vi "Handle Player.vi"(6 "Move Queue Element":T1, 7 "Move in":T4={"InPlayPos Dict"=variant(i32[] [])}, 8 "error in (no error)":errorcluster, 11 "Maze 2.0 in":refnum<class "SquareBattle.lvclass">) -> (0 "error out":errorcluster, 3 "Maze 2.0 out":refnum<class "SquareBattle.lvclass">, 5 "Move out":T4={"InPlayPos Dict"=variant(i32[] [])})   [LabVIEW 2014, in "SquareBattle.lvclass"]
uses:
  SquareBattle.lvclass
  Move State Cluster.ctl
  Move Queue Element Cluster.ctl
  Runner/Runner.lvclass
  Action Enum.ctl
  Direction Enum.ctl
  SquareBattle.lvclass/SquareBattle.ctl
  Runner Cluster.ctl
panel:
  # "NOTICE - YOU MUST NOT REMOVE THIS NOTICE. PER THE FOLLOWING LICENSE, YOU MAY REPRODUCE THIS SOFTWARE PROVIDED YOU FOLLOW THE TERMS\nOF THE LICENSE.\n\n---BEGIN BSD LICENSE (http://opensource.org/licenses/BSD-2-Clause)---\nCopyright (c) 2015, Endigit, Inc. <robert@endigit.com>\nAll rights reserved.\n\nRedistribution and use in source and binary forms, with or without modification, are permitted provided that the following conditions are met:\n\n1. Redistributions of source code must retain the above copyright notice, this list of conditions and the following disclaimer.\n\n2. Redistributions in binary form must reproduce the above copyright notice, this list of conditions and the following disclaimer in the documentation and/or other \nmaterials provided with the distribution.\n\nTHIS SOFTWARE IS PROVIDED BY THE COPYRIGHT HOLDERS AND CONTRIBUTORS \"AS IS\" AND ANY EXPRESS OR IMPLIED WARRANTIES, INCLUDING, BUT NOT \nLIMITED TO, THE IMPLIED WARRANTIES OF MERCHANTABILITY AND FITNESS FOR A PARTICULAR PURPOSE ARE DISCLAIMED. IN NO EVENT SHALL THE COPYRIGHT \nHOLDER OR CONTRIBUTORS BE LIABLE FOR ANY DIRECT, INDIRECT, INCIDENTAL, SPECIAL, EXEMPLARY, OR CONSEQUENTIAL DAMAGES (INCLUDING, BUT NOT \nLIMITED TO, PROCUREMENT OF SUBSTITUTE GOODS OR SERVICES; LOSS OF USE, DATA, OR PROFITS; OR BUSINESS INTERRUPTION) HOWEVER CAUSED AND ON \nANY THEORY OF LIABILITY, WHETHER IN CONTRACT, STRICT LIABILITY, OR TORT (INCLUDING NEGLIGENCE OR OTHERWISE) ARISING IN ANY WAY OUT OF THE USE \nOF THIS SOFTWARE, EVEN IF ADVISED OF THE POSSIBILITY OF SUCH DAMAGE.\n---END BSD LICENSE---"
  # "What information:\n\nfor in play squares:\nID of players in square\nIs attacked."
  # "What information:\n\nfor in play squares:\nID of players in square\nIs attacked."
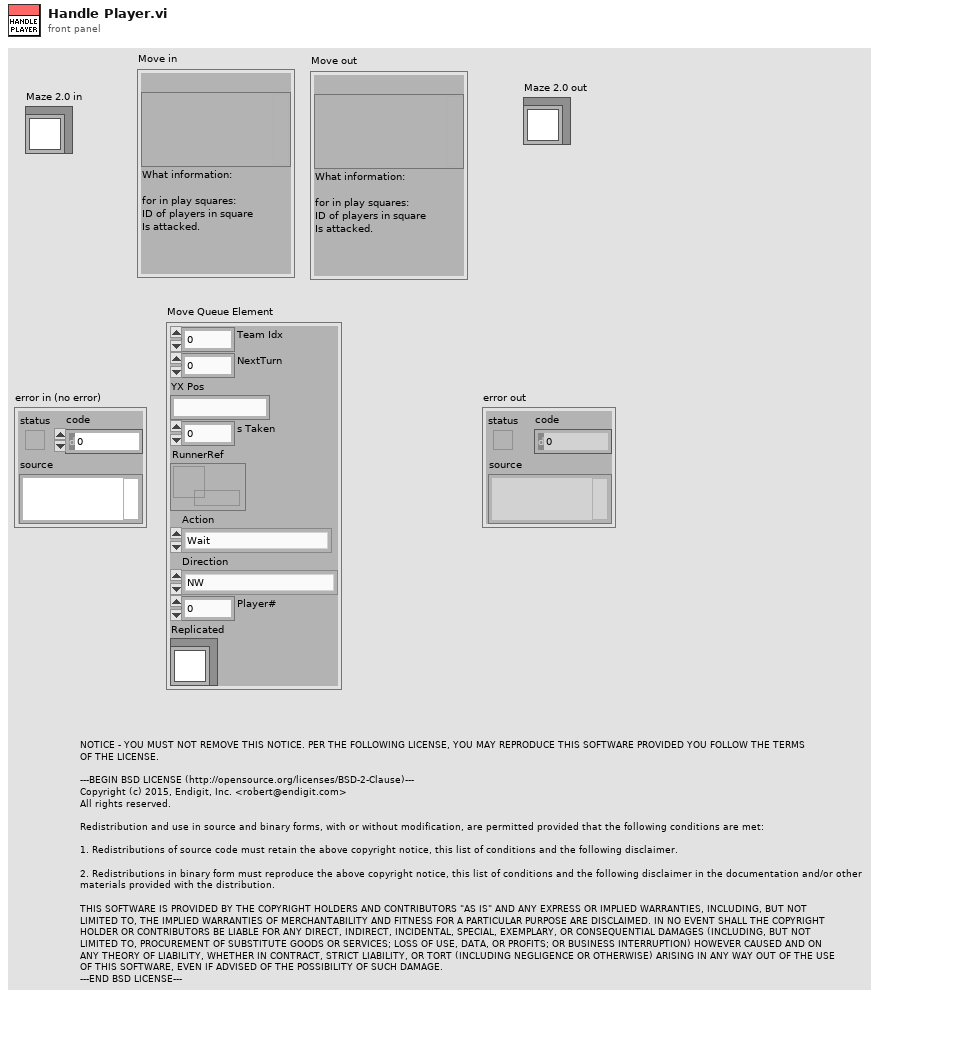
[diagram p1: front panel]
types:
  T1 = typedef "SquareBattle.lvclass/Move Queue Element Cluster.ctl" = cluster{"Team Idx":i32, "NextTurn":u32, "YX Pos":string, "s Taken":dbl, "RunnerRef":refnum<data-value>, "Action":T2, "Direction":T3, "Player#":i32, "Replicated":refnum<class "Runner.lvclass">}
  T2 = typedef "SquareBattle.lvclass/Action Enum.ctl" = enum16{"Wait", "Move", "Attack", "Replicate"}
  T3 = typedef "SquareBattle.lvclass/Direction Enum.ctl" = enum16{"NW", "N", "NE", "E", "SE", "S", "SW", "W"}
  T4 = typedef "SquareBattle.lvclass/Move State Cluster.ctl" = cluster{"InPlayPos Dict":variant}
  T5 = typedef "SquareBattle.lvclass/Runner Cluster.ctl" = cluster{"Attacked?":bool, "RunnerRef":refnum<data-value>, "TeamIdx":i32, "Player #":i32, "NextPlay":u32}
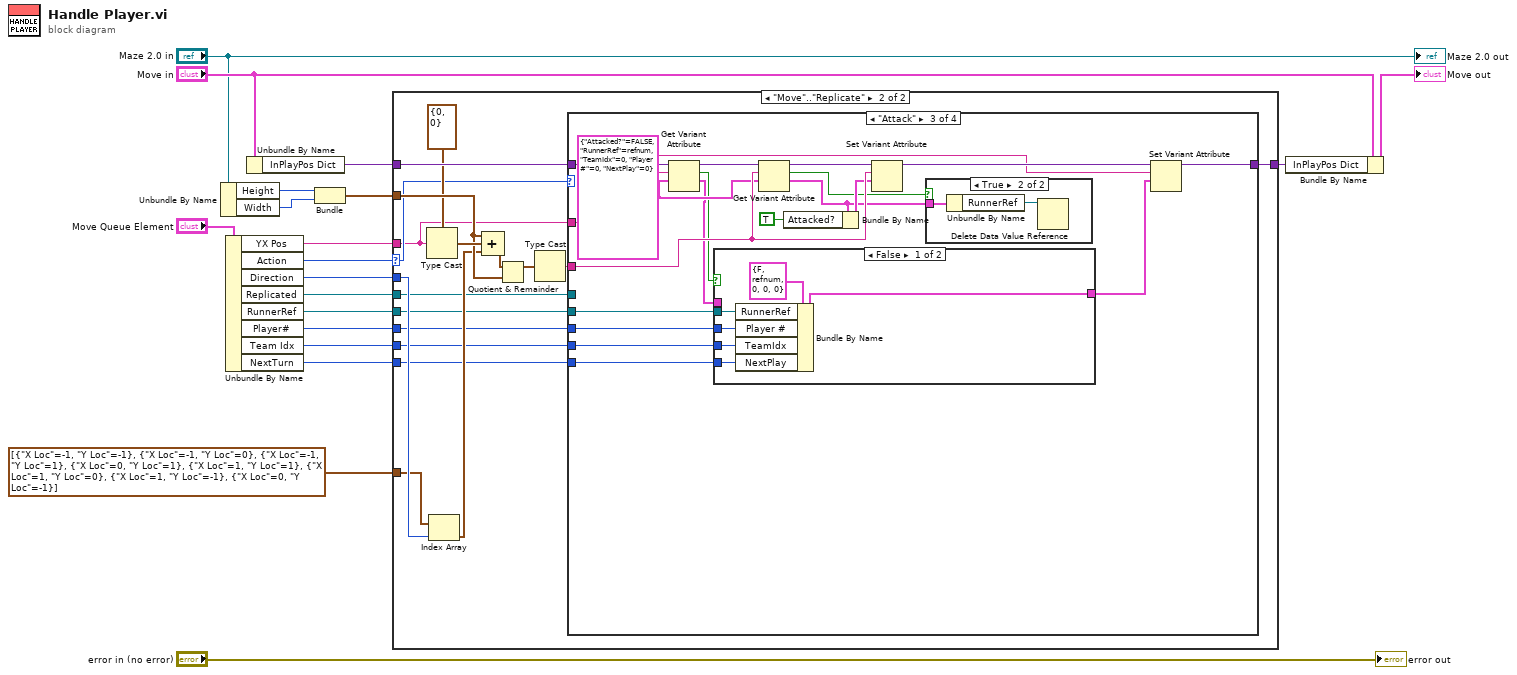
[diagram p0: block diagram]
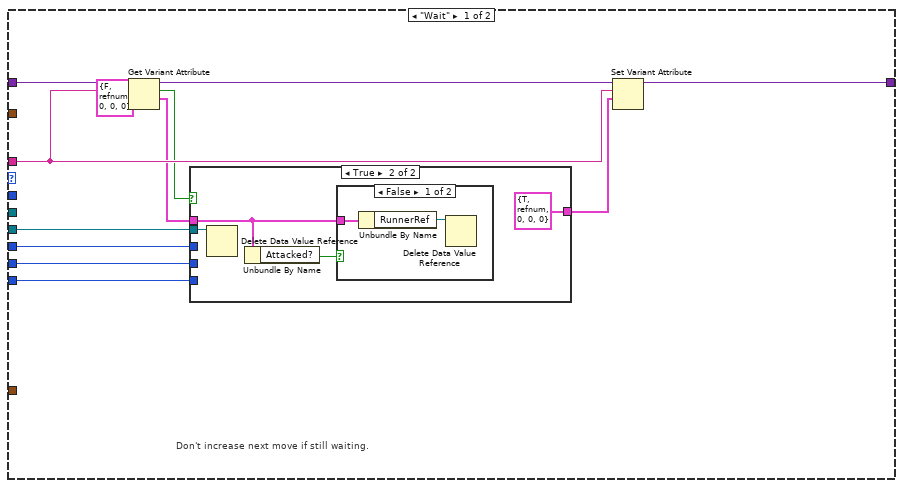
[diagram p2: hidden frame]
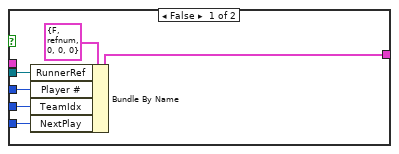
[diagram p3: hidden frame]
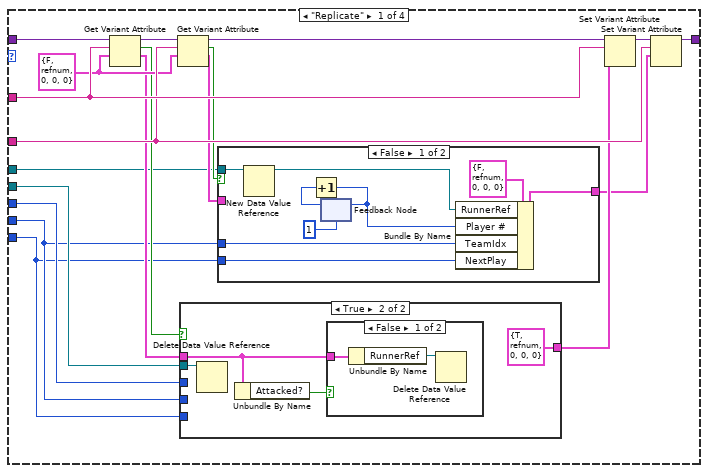
[diagram p5: hidden frame]
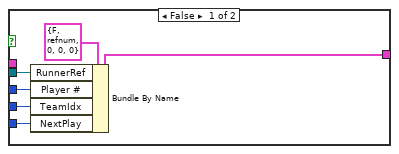
[diagram p6: hidden frame]
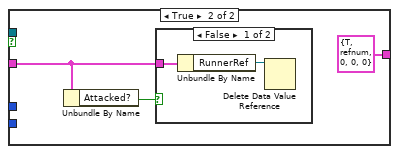
[diagram p8: hidden frame]
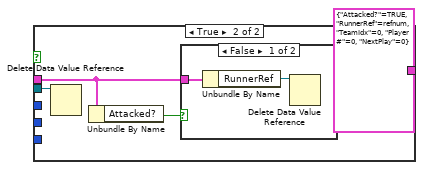
[diagram p12: hidden frame]
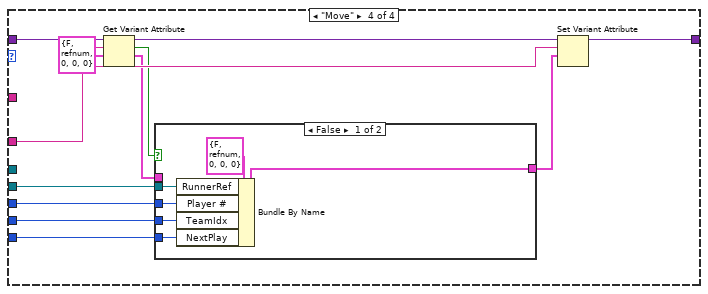
[diagram p14: hidden frame]
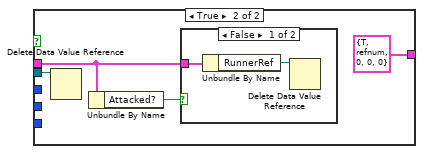
[diagram p15: hidden frame]
diagram:
  n1 = Unbundle By Name("Maze 2.0 in") -> ("Height"=w9:i32, "Width"=w8:i32)
  n2 = Unbundle By Name("Move Queue Element") -> ("YX Pos"=w13:string, "Action"=w12:T2, "Direction"=w16:T3, "Replicated"=w15:refnum<class "Runner.lvclass">, "RunnerRef"=w5:refnum<data-value>, "Player#"=w4:i32, "Team Idx"=w2:i32, "NextTurn"=w1:u32)
  n3 = Unbundle By Name("Move in") -> ("InPlayPos Dict"=w14:variant)
  n4 = Bundle("Height"=w9, "Width"=w8) -> (w7:cluster{"Height":i32, "Width":i32})  [unwired: 1 in]
  n5 = case shown="\"Move\"..\"Replicate\"" w12 {
    selector: w12 -> [_ w51]
    tunnel: w16 -> [_ w55]
    tunnel: w15 -> [_ w47]
    tunnel: w14 -> [w31 w61]
    tunnel: w13 -> [w24 w50]
    tunnel: w2 -> [w30 w49]
    tunnel: [w28 w46] -> w11
    tunnel: w7 -> [_ w57]
    tunnel: cluster{"X Loc":i32, "Y Loc":i32}[] [{"X Loc"=-1, "Y Loc"=-1}, {"X Loc"=-1, "Y Loc"=0}, {"X Loc"=-1, "Y Loc"=1}, {"X Loc"=0, "Y Loc"=1}, {"X Loc"=1, "Y Loc"=1}, {"X Loc"=1, "Y Loc"=0}, {"X Loc"=1, "Y Loc"=-1}, {"X Loc"=0, "Y Loc"=-1}] -> [_ w54]
    tunnel: w1 -> [w27 w48]
    tunnel: w5 -> [w26 w45]
    tunnel: w4 -> [w25 w44]
    frame "Wait" {
      # "Don't increase next move if still waiting."
      n6 = Get Variant Attribute(Variant=w31, name=w24, default value (empty Variant)=T5 {"Attacked?"=FALSE, "RunnerRef"=refnum, "TeamIdx"=0, "Player #"=0, "NextPlay"=0} ("Cluster")) -> (duplicate Variant=w29:variant, found=w22:bool, value=w20:T5)  [unwired: 1 in, 1 out]
      n7 = case shown="True" w22 {
        tunnel: w30 -> [w37 _]
        tunnel: w27 -> [w36 _]
        tunnel: w26 -> [w35 w38]
        tunnel: w25 -> [w34 _]
        tunnel: [w32 T5 {"Attacked?"=TRUE, "RunnerRef"=refnum, "TeamIdx"=0, "Player #"=0, "NextPlay"=0} ("Cluster")] -> w21
        tunnel: w20 -> [_ w39]
        frame False {
          n8 = Bundle By Name(cluster=T5 {"Attacked?"=FALSE, "RunnerRef"=refnum, "TeamIdx"=0, "Player #"=0, "NextPlay"=0} ("Cluster"), "RunnerRef"=w35, "Player #"=w34, "TeamIdx"=w37, "NextPlay"=w36) -> (w32:T5)
        }
        frame True {
          n9 = Delete Data Value Reference(data value reference=w38) -> ()  [unwired: 1 in, 2 out]
          n10 = Unbundle By Name(w39) -> ("Attacked?"=w40:bool)
          n11 = case shown="False" w40 {
            tunnel: w39 -> [w43 _]
            frame False {
              n12 = Unbundle By Name(w43) -> ("RunnerRef"=w42:refnum<data-value>)
              n13 = Delete Data Value Reference(data value reference=w42) -> ()  [unwired: 1 in, 2 out]
            }
            frame True {
            }
          }
        }
      }
      n14 = Set Variant Attribute(Variant=w29, name=w24, value=w21) -> (Variant out=w28:variant)  [unwired: 1 in, 2 out]
    }
    frame "Move".."Replicate" {
      n15 = Type Cast(type=cluster{"Y":i32, "X":i32} {"Y"=0, "X"=0}, x=w50) -> (*(type *) &x=w59:cluster{"Y":i32, "X":i32})
      n16 = Index Array(array=w54, index=w55) -> (element=w53:cluster{"X Loc":i32, "Y Loc":i32})
      n17 = Compound Arithmetic op=ADD(w57, w59, w53) -> (w60:cluster{i32, i32})
      n18 = Quotient & Remainder(x=w60, y=w57) -> (x-y*floor(x/y)=w58:cluster{i32, i32})  [unwired: 1 out]
      n19 = Type Cast(x=w58) -> (*(type *) &x=w52:string)  [unwired: 1 in]
      n20 = case shown="\"Attack\"" w51 {
        tunnel: w61 -> [w80 w107 w126 w149]
        tunnel: w52 -> [w74 _ w123 w151]
        tunnel: w50 -> [w77 _ w110 _]
        tunnel: w49 -> [w63 _ w115 w143]
        tunnel: w48 -> [w62 _ w114 w142]
        tunnel: w47 -> [w65 _ _ _]
        tunnel: [w75 w107 w112 w152] -> w46
        tunnel: w45 -> [w70 _ w118 w147]
        tunnel: w44 -> [w69 _ w116 w144]
        frame "Replicate" {
          w73 = T5 {"Attacked?"=FALSE, "RunnerRef"=refnum, "TeamIdx"=0, "Player #"=0, "NextPlay"=0} ("Cluster")
          n21 = Get Variant Attribute(Variant=w80, name=w77, default value (empty Variant)=w73) -> (duplicate Variant=w79:variant, found=w72:bool, value=w71:T5)  [unwired: 1 in, 1 out]
          n22 = Get Variant Attribute(Variant=w79, name=w74, default value (empty Variant)=w73) -> (duplicate Variant=w78:variant, found=w67:bool, value=w66:T5)  [unwired: 1 in, 1 out]
          n23 = case shown="True" w72 {
            tunnel: w63 -> [w86 _]
            tunnel: w62 -> [w85 _]
            tunnel: w70 -> [w84 w87]
            tunnel: w69 -> [w83 _]
            tunnel: [w81 T5 {"Attacked?"=TRUE, "RunnerRef"=refnum, "TeamIdx"=0, "Player #"=0, "NextPlay"=0} ("Cluster")] -> w68
            tunnel: w71 -> [_ w88]
            frame False {
              n24 = Bundle By Name(cluster=T5 {"Attacked?"=FALSE, "RunnerRef"=refnum, "TeamIdx"=0, "Player #"=0, "NextPlay"=0} ("Cluster"), "RunnerRef"=w84, "Player #"=w83, "TeamIdx"=w86, "NextPlay"=w85) -> (w81:T5)
            }
            frame True {
              n25 = Delete Data Value Reference(data value reference=w87) -> ()  [unwired: 1 in, 2 out]
              n26 = Unbundle By Name(w88) -> ("Attacked?"=w89:bool)
              n27 = case shown="False" w89 {
                tunnel: w88 -> [w92 _]
                frame False {
                  n28 = Unbundle By Name(w92) -> ("RunnerRef"=w91:refnum<data-value>)
                  n29 = Delete Data Value Reference(data value reference=w91) -> ()  [unwired: 1 in, 2 out]
                }
                frame True {
                }
              }
            }
          }
          n30 = case shown="False" w67 {
            tunnel: w63 -> [w101 _]
            tunnel: w62 -> [w100 _]
            tunnel: [w98 T5 {"Attacked?"=TRUE, "RunnerRef"=refnum, "TeamIdx"=0, "Player #"=0, "NextPlay"=0} ("Cluster")] -> w64
            tunnel: w66 -> [_ w102]
            tunnel: w65 -> [w96 _]
            frame False {
              n31 = New Data Value Reference(data value=w96) -> (data value reference=w97:refnum<data-value>)  [unwired: 1 in, 1 out]
              n32 = feedback #1(1) -> (w95:i32)
              n33 = Increment(x=w95) -> (x+1=w93:i32)
              n34 = feedback-in #1(w93) -> ()
              n35 = Bundle By Name(cluster=T5 {"Attacked?"=FALSE, "RunnerRef"=refnum, "TeamIdx"=0, "Player #"=0, "NextPlay"=0} ("Cluster"), "RunnerRef"=w97, "Player #"=w93, "TeamIdx"=w101, "NextPlay"=w100) -> (w98:T5)
            }
            frame True {
              n36 = Unbundle By Name(w102) -> ("Attacked?"=w103:bool)
              n37 = case shown="False" w103 {
                tunnel: w102 -> [w106 _]
                frame False {
                  n38 = Unbundle By Name(w106) -> ("RunnerRef"=w105:refnum<data-value>)
                  n39 = Delete Data Value Reference(data value reference=w105) -> ()  [unwired: 1 in, 2 out]
                }
                frame True {
                }
              }
            }
          }
          n40 = Set Variant Attribute(Variant=w78, name=w77, value=w68) -> (Variant out=w76:variant)  [unwired: 1 in, 2 out]
          n41 = Set Variant Attribute(Variant=w76, name=w74, value=w64) -> (Variant out=w75:variant)  [unwired: 1 in, 2 out]
        }
        frame "Wait" {
          # "shouldn't ever get here..."
        }
        frame "Attack" {
          w120 = T5 {"Attacked?"=FALSE, "RunnerRef"=refnum, "TeamIdx"=0, "Player #"=0, "NextPlay"=0} ("Cluster")
          n42 = Get Variant Attribute(Variant=w126, name=w110, default value (empty Variant)=w120) -> (duplicate Variant=w125:variant, found=w119:bool, value=w117:T5)  [unwired: 1 in, 1 out]
          n43 = case shown="False" w119 {
            tunnel: w115 -> [w134 _]
            tunnel: w114 -> [w133 _]
            tunnel: w118 -> [w132 w135]
            tunnel: w116 -> [w131 _]
            tunnel: [w129 T5 {"Attacked?"=TRUE, "RunnerRef"=refnum, "TeamIdx"=0, "Player #"=0, "NextPlay"=0} ("Cluster")] -> w111
            tunnel: w117 -> [_ w136]
            frame False {
              n44 = Bundle By Name(cluster=T5 {"Attacked?"=FALSE, "RunnerRef"=refnum, "TeamIdx"=0, "Player #"=0, "NextPlay"=0} ("Cluster"), "RunnerRef"=w132, "Player #"=w131, "TeamIdx"=w134, "NextPlay"=w133) -> (w129:T5)
            }
            frame True {
              n45 = Delete Data Value Reference(data value reference=w135) -> ()  [unwired: 1 in, 2 out]
              n46 = Unbundle By Name(w136) -> ("Attacked?"=w137:bool)
              n47 = case shown="False" w137 {
                tunnel: w136 -> [w140 _]
                frame False {
                  n48 = Unbundle By Name(w140) -> ("RunnerRef"=w139:refnum<data-value>)
                  n49 = Delete Data Value Reference(data value reference=w139) -> ()  [unwired: 1 in, 2 out]
                }
                frame True {
                }
              }
            }
          }
          n50 = Get Variant Attribute(Variant=w125, name=w123, default value (empty Variant)=w120) -> (duplicate Variant=w124:variant, found=w108:bool, value=w109:T5)  [unwired: 1 in, 1 out]
          n51 = Bundle By Name(cluster=w109, "Attacked?"=TRUE) -> (w122:T5)
          n52 = Set Variant Attribute(Variant=w124, name=w123, value=w122) -> (Variant out=w113:variant)  [unwired: 1 in, 2 out]
          n53 = case shown="True" w108 {
            tunnel: w109 -> [_ w128]
            frame False {
            }
            frame True {
              n54 = Unbundle By Name(w128) -> ("RunnerRef"=w127:refnum<data-value>)
              n55 = Delete Data Value Reference(data value reference=w127) -> ()  [unwired: 1 in, 2 out]
            }
          }
          n56 = Set Variant Attribute(Variant=w113, name=w110, value=w111) -> (Variant out=w112:variant)  [unwired: 1 in, 2 out]
        }
        frame "Move" {
          n57 = Get Variant Attribute(Variant=w149, name=w151, default value (empty Variant)=T5 {"Attacked?"=FALSE, "RunnerRef"=refnum, "TeamIdx"=0, "Player #"=0, "NextPlay"=0} ("Cluster")) -> (duplicate Variant=w150:variant, found=w146:bool, value=w145:T5)  [unwired: 1 in, 1 out]
          n58 = case shown="False" w146 {
            tunnel: w143 -> [w158 _]
            tunnel: w142 -> [w157 _]
            tunnel: w147 -> [w156 w159]
            tunnel: w144 -> [w155 _]
            tunnel: [w153 T5 {"Attacked?"=TRUE, "RunnerRef"=refnum, "TeamIdx"=0, "Player #"=0, "NextPlay"=0} ("Cluster")] -> w141
            tunnel: w145 -> [_ w160]
            frame False {
              n59 = Bundle By Name(cluster=T5 {"Attacked?"=FALSE, "RunnerRef"=refnum, "TeamIdx"=0, "Player #"=0, "NextPlay"=0} ("Cluster"), "RunnerRef"=w156, "Player #"=w155, "TeamIdx"=w158, "NextPlay"=w157) -> (w153:T5)
            }
            frame True {
              n60 = Delete Data Value Reference(data value reference=w159) -> ()  [unwired: 1 in, 2 out]
              n61 = Unbundle By Name(w160) -> ("Attacked?"=w161:bool)
              n62 = case shown="False" w161 {
                tunnel: w160 -> [w164 _]
                frame False {
                  n63 = Unbundle By Name(w164) -> ("RunnerRef"=w163:refnum<data-value>)
                  n64 = Delete Data Value Reference(data value reference=w163) -> ()  [unwired: 1 in, 2 out]
                }
                frame True {
                }
              }
            }
          }
          n65 = Set Variant Attribute(Variant=w150, name=w151, value=w141) -> (Variant out=w152:variant)  [unwired: 1 in, 2 out]
        }
      }
    }
  }
  n66 = Bundle By Name(cluster="Move in", "InPlayPos Dict"=w11) -> (→"Move out":T4)
  "error out" <- "error in (no error)"
  "Maze 2.0 out" <- "Maze 2.0 in"
